vi "Updatevalue.vi"(0 "ParameterConf in":refnum<class "ParameterConf.lvclass">, 1 "CONTROL PWM":T1, 2 "PARA":cluster{"STEP":i16, "FEEDRATE":dbl}, 3 "error in (no error)":errorcluster) -> (7 "ParameterConf out":refnum<class "ParameterConf.lvclass">, 10 "error out":errorcluster)   [LabVIEW 2014, in "LibraryGcode.lvlib" / "ParameterConf.lvclass"]
uses:
  ParameterConf.lvclass
  ParameterConf.lvclass/ParameterConf.ctl
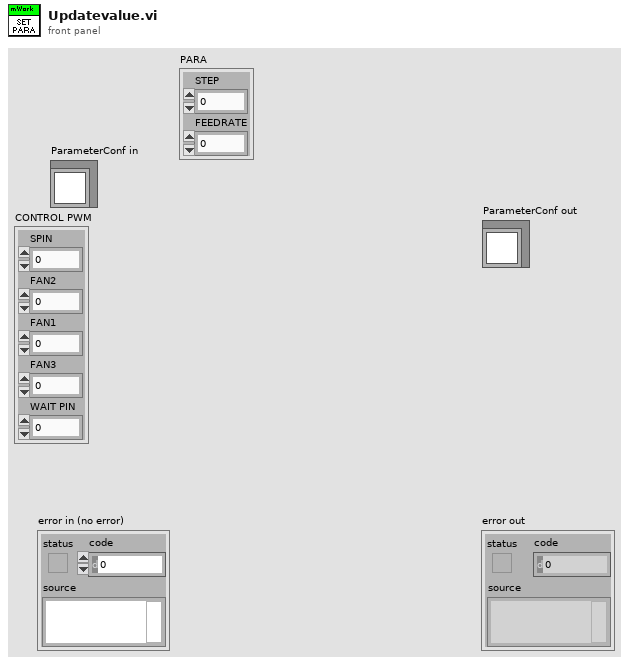
[diagram p1: front panel]
types:
  T1 = cluster{"SPIN":dbl, "FAN2":dbl, "FAN1":dbl, "FAN3":dbl, "WAIT PIN ":dbl}
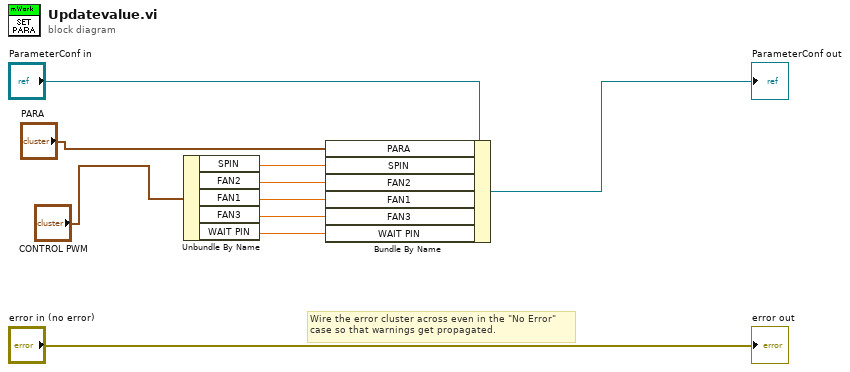
[diagram p0: block diagram]
diagram:
  # "Wire the error cluster across even in the \"No Error\"\ncase so that warnings get propagated."
  n1 = Unbundle By Name("CONTROL PWM") -> ("SPIN"=w5:dbl, "FAN2"=w4:dbl, "FAN1"=w3:dbl, "FAN3"=w2:dbl, "WAIT PIN"=w1:dbl)
  n2 = Bundle By Name(cluster="ParameterConf in", "PARA"="PARA", "SPIN"=w5, "FAN2"=w4, "FAN1"=w3, "FAN3"=w2, "WAIT PIN"=w1) -> (→"ParameterConf out":refnum<class "ParameterConf.lvclass">)
  "error out" <- "error in (no error)"
